vi "SetGasIndex.vi"(7 "Timeout (ms)":u32=2000, 8 "Error In":errorcluster, 10 "Gas Index":u16=1 min=1 max=10 step=1, 11 "Sierra M100 In":refnum<visa-resource-name>) -> (0 "Error Out":errorcluster, 2 "Set?":bool, 3 "Sierra M100 Out":refnum<visa-resource-name>)   [LabVIEW 2012, in "Sierra-M100.lvlib"]
doc: "This VI sets the gas index (1-10). The gas index is an indicator of the calibrated gas for the mass flow controller. Use \"Set Gas\" VI instead."
uses:
  Sierra-M100.lvlib
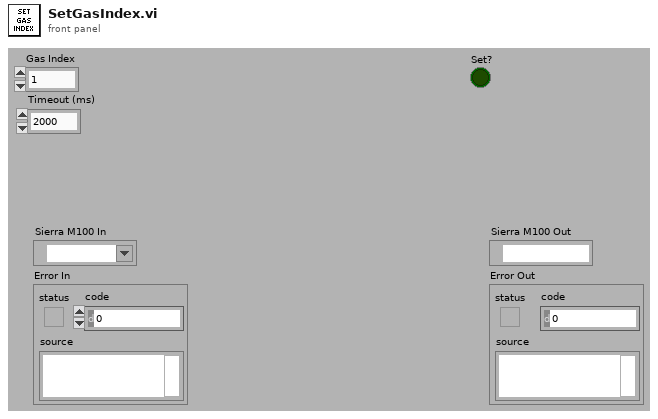
[diagram p1: front panel]
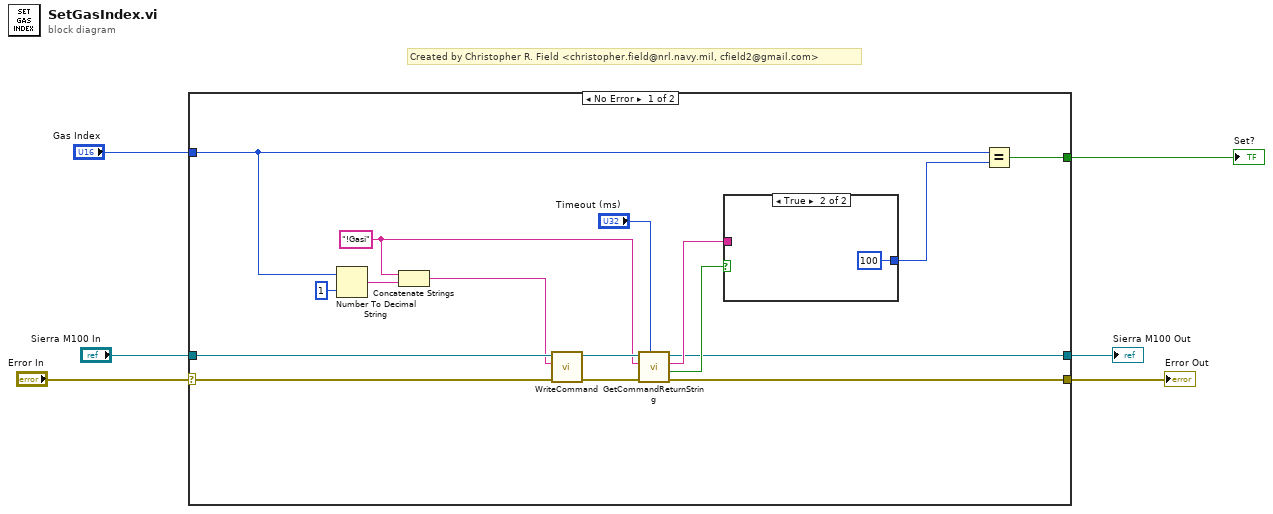
[diagram p0: block diagram]
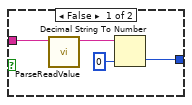
[diagram p2: hidden frame]
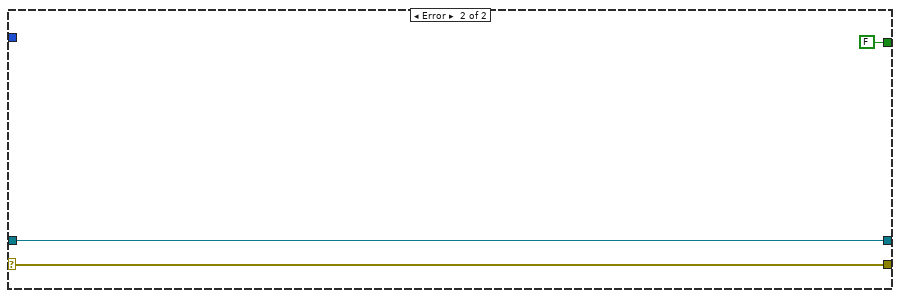
[diagram p3: hidden frame]
diagram:
  # "Created by Christopher R. Field <christopher.field@nrl.navy.mil, cfield2@gmail.com>"
  n1 = case shown="No Error" "Error In" {
    selector: "Error In" -> [w7 w30]
    tunnel: "Sierra M100 In" -> [w20 w29]
    tunnel: [w12 w29] -> w5
    tunnel: [w11 w30] -> w4
    tunnel: "Gas Index" -> [w9 _]
    tunnel: [w8 FALSE] -> w2
    frame No Error {
      w16 = "!Gasi"
      n2 = Number To Decimal String(number=w9, width (-)=i16 1) -> (decimal integer string=w21:string)
      n3 = Concatenate Strings(w16, w21) -> (w19:string)
      n4 = call "WriteCommand.vi"("Error In"=w7, "Command"=w19, "Smart Trak 2 In"=w20) -> ("Error Out"=w17:errorcluster, "Smart Trak 2 Out"=w18:refnum<visa-resource-name>)  [unwired: 5 in, 2 out]
      n5 = call "GetCommandReturnString.vi"("Timeout (ms)"="Timeout (ms)", "Error In"=w17, "Command"=w16, "Smart Trak 2 In"=w18) -> ("Error Out"=w11:errorcluster, "Timeout?"=w13:bool, "Return String"=w14:string, "Smart Trak 2 Out"=w12:refnum<visa-resource-name>)  [unwired: 4 in]
      n6 = case shown="True" w13 {
        tunnel: w14 -> [w26 _]
        tunnel: [w24 u16 100] -> w10
        frame False {
          n7 = call "ParseReadValue.vi"("Read Buffer"=w26) -> ("Value"=w25:string)  [unwired: 10 in]
          n8 = Decimal String To Number(string=w25, default (0L)=u16 0 ("default (0 I32)")) -> (number=w24:u16)  [unwired: 1 in, 1 out]
        }
        frame True {
        }
      }
      n9 = Equal?(x=w9, y=w10) -> (x = y?=w8:bool)
    }
    frame Error {
    }
  }
  "Sierra M100 Out" <- w5
  "Error Out" <- w4
  "Set?" <- w2
